vi "BlueTooth Sound Input.vi"(8 "error in":errorcluster={"status"=FALSE, "code"=1073676294, "source"="CommunicationTool.vi:3540001->TestSequenceSubVI.vi:4310001->SequenceVI.vi:6750002->AVN TestSystem.vi中的VISA读取"} caption="错误输入（无错误）") -> (0 "error out":errorcluster caption="错误输出", 3 "Raw Data 3":waveform(dbl)(graph)={"t0"=timestamp(3484094375.46875 s since 1904-01-01), "dt"=2.5e-05, "Y"=array[80000 elements]}, 11 "Device ID":u32 format="%.0x")   [LabVIEW 2013]
doc: "This VI illustrates how to acquire sound samples continuously from a specified device. It requires the use of a microphone attached to the sound card. You can specify the number of samples to acquire, sample rate, number of channels and a bit rate per sample. The VI also plots the raw data as the acquisition is made."
uses:
  <vilib>/sound2/lvsound2.llb/Sampling Mode.ctl
  <vilib>/sound2/lvsound2.llb/Sound Data Format.ctl
  <vilib>/registry/registry.llb/Registry SAM.ctl
  <vilib>/registry/registry.llb/Registry RtKey.ctl
  <vilib>/registry/registry.llb/Read Registry Value Simple STR.vi
  <vilib>/sound2/lvsound2.llb/Sound Input Read (DBL).vi
  <vilib>/Waveform/WDTOps.llb/WDT Index Channel DBL.vi
  <vilib>/Waveform/WDTOps.llb/WDT Get Waveform Subset DBL.vi
  <vilib>/measure/macond.llb/FIR Filter for 1 Chan.vi
  <vilib>/measure/matone.llb/Extract Single Tone Information 1 Chan.vi
  <vilib>/measure/NI_MAPro.lvlib
panel:
  out "String/Binary data":string="Bluetooth Audio" caption="Device"
  out "frequency":dbl=999.8807274260902 caption="检测到的频率" format="%.2p"
  out "amplitude":dbl=0.457250871853994 caption="检测到的幅值" format="%.2p"
  out "Raw Data":waveform(dbl)[](graph)=[{"t0"=timestamp(3484094373.46875 s since 1904-01-01), "dt"=2.5e-05, "Y"=array[160000 elements]}, {"t0"=timestamp(3484094373.46875 s since 1904-01-01), "dt"=2.5e-05, "Y"=array[160000 elements]}]
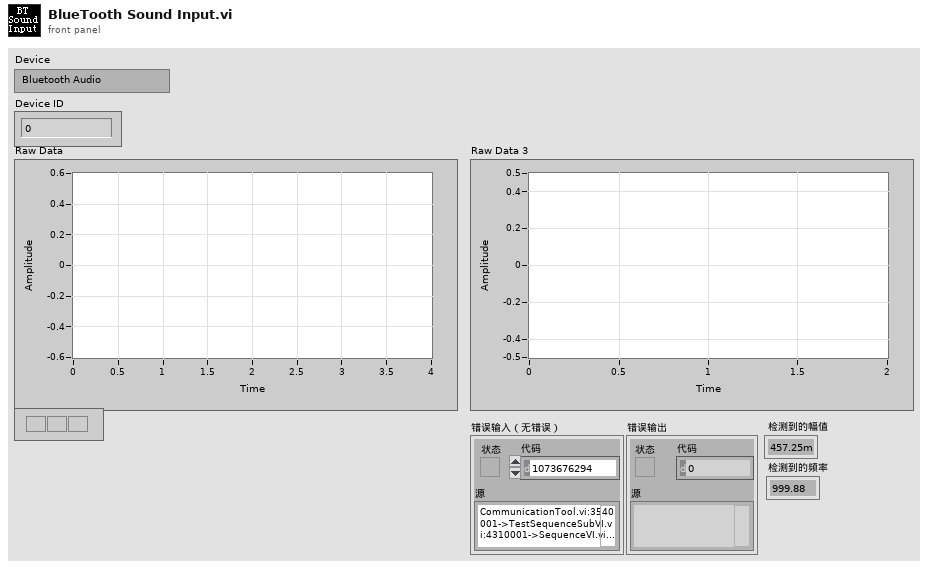
[diagram p1: front panel]
types:
  T1 = typedef "Registry RtKey.ctl" = enum32{"HKEY_CLASSES_ROOT", "HKEY_CURRENT_USER", "HKEY_LOCAL_MACHINE", "HKEY_USERS", "HKEY_PERFORMANCE_DATA", "HKEY_CURRENT_CONFIG", "HKEY_DYN_DATA"}
  T2 = typedef "Registry SAM.ctl" = enum32{"KEY_QUERY_VALUE", "KEY_SET_VALUE", "KEY_CREATE_SUB_KEY", "KEY_ENUMERATE_SUB_KEYS", "KEY_NOTIFY", "KEY_CREATE_LINK", "KEY_READ", "KEY_WRITE", "KEY_ALL_ACCESS", "KEY_READ | KEY_WRITE"}
  T3 = cluster{"Topology":enum16{"Off", "FIR by Specification", "Equi-ripple FIR", "Windowed FIR"}, "Type":enum16{"Lowpass", "Highpass", "Bandpass", "Bandstop"}, "#Taps":i32, "Lower PB":dbl, "Upper PB":dbl, "Lower SB":dbl, "Upper SB":dbl}
  T4 = typedef "Sound Data Format.ctl" = cluster{"sample rate (S/s)":dbl, "number of channels":i32, "bits per sample":i32}
  T5 = typedef "Sampling Mode.ctl" = i32
  T6 = typedef "Registry refnum.ctl" = refnum<k1>
  T7 = typedef "Sound Input Task ID.ctl" = u32
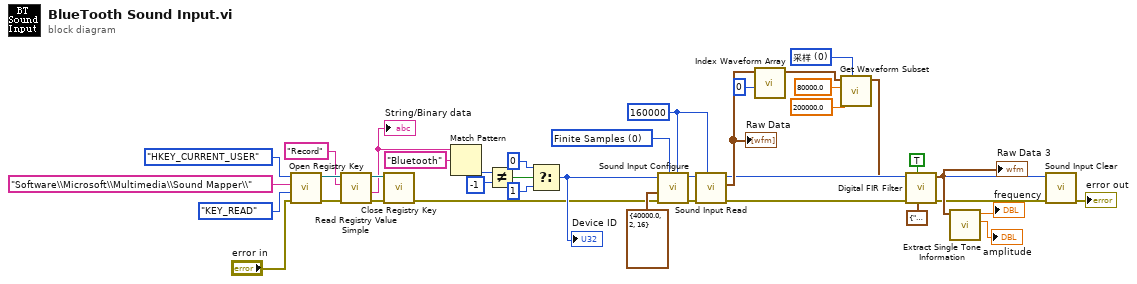
[diagram p0: block diagram]
diagram:
  w38 = 160000 ("Number of Samples/ch")
  w29 = u16 0 items=["采样", "相对时间"] ("start/duration format")
  w39 = T5 0 items=["Finite Samples", "Continuous Samples"] ("sample mode")
  n1 = call <vilib>:"Open Registry Key.vi"("error in (no error)"="error in", "security access mask (KEY_READ | KEY_WRITE)"=Registry_SAM."KEY_READ", "subkey"="Software\\Microsoft\\Multimedia\\Sound Mapper\\", "root key (HKEY_LOCAL_MACHINE)"=Registry_RtKey."HKEY_CURRENT_USER") -> ("error out"=w14:errorcluster, "refnum out"=w18:T6)  [unwired: 6 out]
  n2 = call-poly <vilib>:"Read Registry Value Simple.vi"("error in (no error)"=w14, "value"="Record", "refnum"=w18) -> ("error out"=w13:errorcluster, "String/Binary data"=w10:string, "refnum out"=w12:T6)  [unwired: 1 in, 3 out]
  "String/Binary data" <- w10
  n3 = call <vilib>:"Close Registry Key.vi"("error in (no error)"=w13, "refnum"=w12) -> ("error out"=w2:errorcluster)  [unwired: 5 out]
  n4 = Match Pattern(string=w10, regular expression="Bluetooth" ("正则表达式")) -> (offset past match=w8:i32)  [unwired: 1 in, 3 out]
  n5 = Not Equal?(x=w8, y=-1) -> (x != y?=w6:bool)
  n6 = Select(t=u32 0 ("Device ID 2"), s=w6, f=u32 1 ("Device ID 2")) -> (s? t:f=w3:u32)
  "Device ID" <- w3
  n7 = call <vilib>:"Sound Input Configure.vi"("number of samples/ch"=w38, "sample mode"=w39, "error in (no error)"=w2, "sound format"=T4 {"sample rate (S/s)"=40000.0, "number of channels"=2, "bits per sample"=16} ("Sound Format"), "device ID"=w3) -> ("error out"=w25:errorcluster, "task ID"=w26:T7)  [unwired: 5 in]
  n8 = call-poly <vilib>:"Sound Input Read.vi"("number of samples/ch"=w38, "error in (no error)"=w25, "task ID"=w26) -> ("error out"=w21:errorcluster, "data"=w34:waveform(dbl)[], "task ID out"=w27:T7)  [unwired: 6 in]
  "Raw Data" <- w34
  n9 = call-poly <vilib>:"Index Waveform Array.vi"("index"=0, "waveform array"=w34) -> ("waveform"=w23:waveform(dbl))  [unwired: 8 in, 1 out]
  n10 = call-poly <vilib>:"Get Waveform Subset.vi"("start/duration format"=w29, "duration"=200000.0, "start samples/time"=80000.0, "waveform in"=w23) -> ("waveform out"=w22:waveform(dbl))  [unwired: 2 in, 3 out]
  n11 = call-poly <vilib>:"Digital FIR Filter.vi"("FIR filter specifications"=T3 {"Topology"=enum."Windowed FIR", "Type"=enum."Bandpass", "#Taps"=200, "Lower PB"=900.0, "Upper PB"=1100.0, "Lower SB"=0.0, "Upper SB"=0.0}, "reset filter"=TRUE, "error in (no error)"=w21, "signal in"=w22) -> ("error out"=w20:errorcluster, "signal out"=w32:waveform(dbl))  [unwired: 5 in, 1 out]
  "Raw Data 3" <- w32
  n12 = call-poly <vilib>:"Extract Single Tone Information.vi"("time signal in"=w32) -> ("detected amplitude"=→"amplitude":dbl, "detected frequency"=→"frequency":dbl)  [unwired: 5 in, 4 out]
  n13 = call <vilib>:"Sound Input Clear.vi"("error in (no error)"=w20, "task ID"=w27) -> ("error out"=→"error out":errorcluster)  [unwired: 9 in]
